vi "NML Bus Scan AH 2500.vi"(3 "error in (no error)":errorcluster {"code" format="%.0x"}, 4 "String Read In":string, 5 "VISA resource name":refnum<visa-resource-name>) -> (0 "error out":errorcluster {"code" format="%.0x"}, 1 "String Read Out":string, 2 "dup VISA Session":refnum<visa-resource-name>)   [LabVIEW 2025]
doc: "Author: Scott Hannahs <sth@magnet.fsu.edu>\n\nThis software is licensed for use under the “MIT License\"\nCopyright (c) 2025 Scott Hannahs, sth@sth@magnet.sthnet.net\n\nPermission is hereby granted, free of charge, to any person obtaining a copy of this software and associated documentation files (the \"Software\"), to deal in the Software without restriction, including without limitation the rights to use, copy, modify, merge, publish, distribute, sublicense, and/or sell copies of the Software, and to permit persons to whom the Software is furnished to do so, subject to the following conditions: The above copyright notice and this permission notice shall be included in all copies or substantial portions of the Software.\n\nTHE SOFTWARE IS PROVIDED \"AS IS\", WITHOUT WARRANTY OF ANY KIND, EXPRESS OR IMPLIED, INCLUDING BUT NOT LIMITED TO THE WARRANTIES OF MERCHANTABILITY, FITNESS FOR A PARTICULAR PURPOSE AND NONINFRINGEMENT. IN NO EVENT SHALL THE AUTHORS OR COPYRIGHT HOLDERS BE LIABLE FOR ANY CLAIM, DAMAGES OR OTHER LIABILITY, WHETHER IN AN ACTION OF CONTRACT, TORT OR OTHERWISE, ARISING FROM, OUT OF OR IN CONNECTION WITH THE SOFTWARE OR THE USE OR OTHER DEALINGS IN THE SOFTWARE."
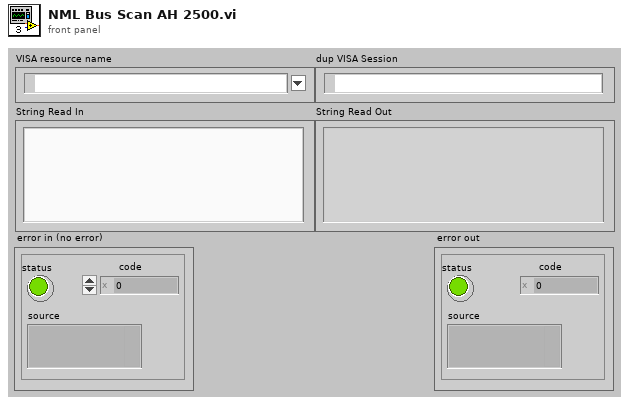
[diagram p1: front panel]
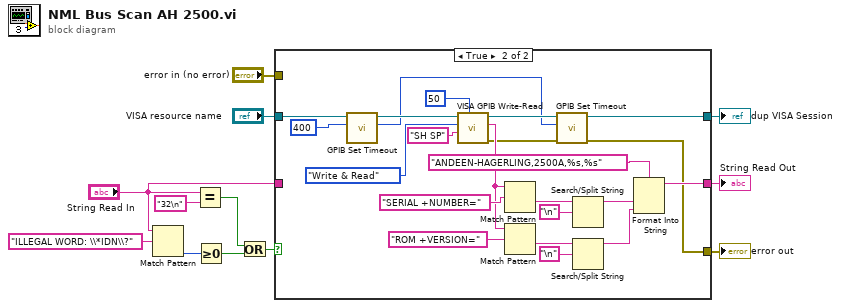
[diagram p0: block diagram]
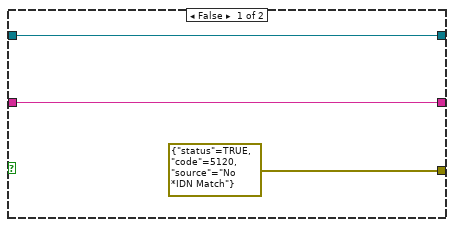
[diagram p2: hidden frame]
diagram:
  n1 = Match Pattern(string="String Read In", regular expression="ILLEGAL WORD: \\*IDN\\?") -> (offset past match=w10:i32)  [unwired: 1 in, 3 out]
  n2 = Equal?(x="String Read In", y="32\n") -> (x = y?=w9:bool)
  n3 = Greater Or Equal To 0?(x=w10) -> (x >= 0?=w7:bool)
  n4 = Or(x=w9, y=w7) -> (x .or. y?=w5:bool)
  n5 = case shown="True" w5 {
    tunnel: [errorcluster {"status"=TRUE, "code"=5120, "source"="No *IDN Match"} ("error out") w17] -> w2
    tunnel: [w15 w26] -> w12
    tunnel: [w14 w16] -> w3
    tunnel: "VISA resource name" -> [w14 w24]
    tunnel: "String Read In" -> [w15 _]
    tunnel: "error in (no error)" -> [_ _]
    frame False {
    }
    frame True {
      n6 = call "GPIB Set Timeout.vi"("Timeout"=u32 400 ("General Settings:Timeout Value"), "VISA resource name"=w24) -> ("Old Timeout"=w20:u32, "dup VISA resource name"=w23:refnum<visa-resource-name>)  [unwired: 3 in, 1 out]
      n7 = call "VISA GPIB Write-Read.vi"("Wait (ms)"=u32 50 ("wait (mS)"), "Command"="SH SP" ("String to Write"), "Action"=enum16{"Write", "Read", "Write & Read"}."Write & Read", "VISA resource name"=w23) -> ("error out"=w19:errorcluster, "String Returned"=w25:string, "dup VISA Session"=w22:refnum<visa-resource-name>)  [unwired: 4 in, 1 out]
      n8 = Match Pattern(string=w25, regular expression="SERIAL +NUMBER=") -> (after substring=w33:string)  [unwired: 1 in, 3 out]
      n9 = Match Pattern(string=w25, regular expression="ROM +VERSION=") -> (after substring=w30:string)  [unwired: 1 in, 3 out]
      n10 = call "GPIB Set Timeout.vi"("Error In"=w19, "Timeout"=w20, "VISA resource name"=w22) -> ("Error Out"=w17:errorcluster, "dup VISA resource name"=w16:refnum<visa-resource-name>)  [unwired: 2 in, 1 out]
      n11 = Search/Split String(string=w33, search string/char (-)="\n") -> (substring before match=w28:string)  [unwired: 1 in, 2 out]
      n12 = Search/Split String(string=w30, search string/char (-)="\n") -> (substring before match=w27:string)  [unwired: 1 in, 2 out]
      n13 = Format Into String(format string="ANDEEN-HAGERLING,2500A,%s,%s", w28, w27) -> (resulting string=w26:string)  [unwired: 2 in, 1 out]
    }
  }
  "String Read Out" <- w12
  "dup VISA Session" <- w3
  "error out" <- w2
